vi "CM_FGV.vi"(7 "FGV_mods":T1=enum."Pulse", 8 "Error In":errorcluster, 11 "DataIn":variant) -> (0 "Error Out":errorcluster, 3 "Rotações":dbl[](array[numeric]))   [LabVIEW 2016]
uses:
  CM_mods.ctl
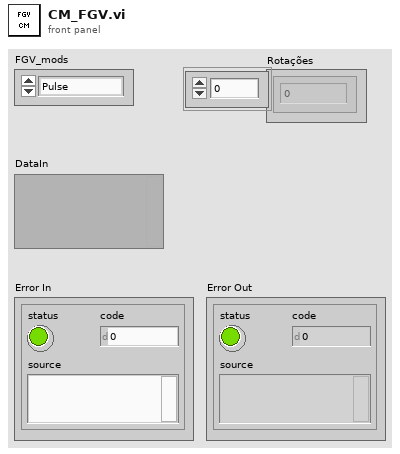
[diagram p1: front panel]
types:
  T1 = typedef "CM_mods.ctl" = enum16{"Init", "Pulse", "Retrieve", "End"}
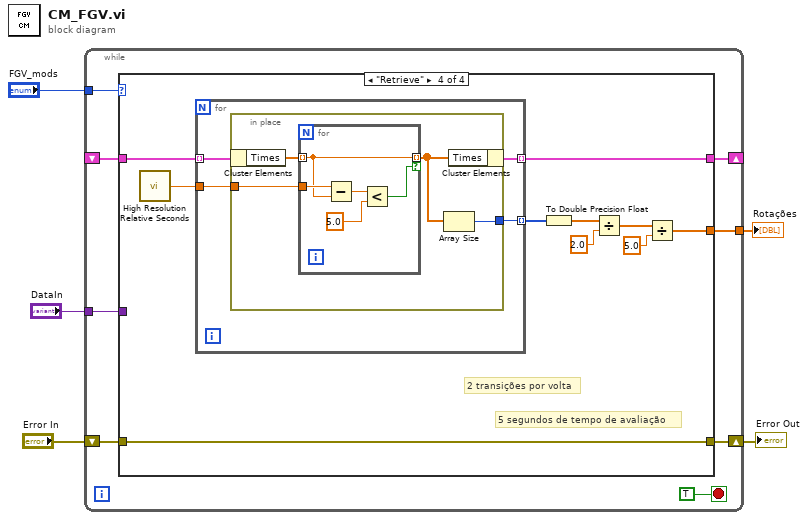
[diagram p0: block diagram]
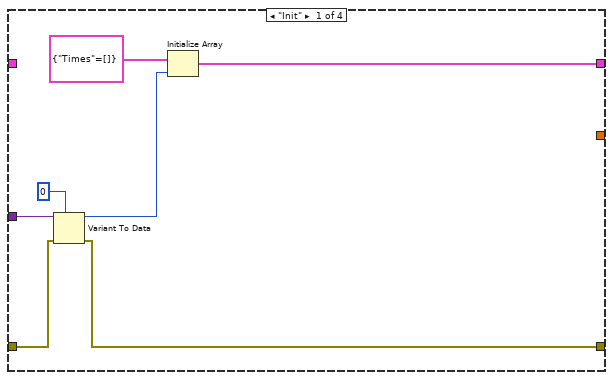
[diagram p2: hidden frame]
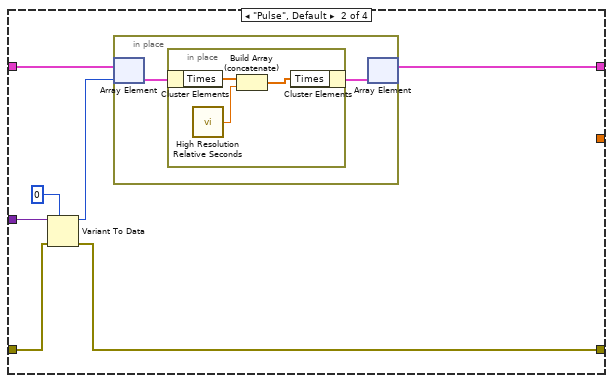
[diagram p3: hidden frame]
diagram:
  n1 = while {
    tunnel: "DataIn" -> [w12]
    tunnel: "FGV_mods" -> [w11]
    shift-right: [w10] -> _
    shift-left: _ -> [w9]
    shift-right: [w7] -> w2
    shift-left: "Error In" -> [w8]
    tunnel: [w6] -> w1
    stop <- TRUE stop-if-true
    n2 = case shown="\"Retrieve\"" w11 {
      tunnel: w12 -> [w20 w26 _ _]
      tunnel: [w16 w21 w34 w42] -> w10
      tunnel: w9 -> [_ w23 w34 w44]
      tunnel: w8 -> [w19 w25 w33 w35]
      tunnel: [w15 w24 w33 w35] -> w7
      tunnel: [_ _ _ w36] -> w6
      frame "Init" {
        n3 = Variant To Data(error in=w19, type=0, Variant=w20) -> (data=w17:i32, error out=w15:errorcluster)
        n4 = Initialize Array(cluster{"Times":dbl[]} {"Times"=[]}, w17) -> (w16:cluster{"Times":dbl[]}[])
      }
      frame "Pulse", Default {
        n5 = Variant To Data(error in=w25, type=0, Variant=w26) -> (data=w22:i32, error out=w24:errorcluster)
        n6 = in-place {
          n7 = in-place-array #1(w23, w22) -> (w29:cluster{"Times":dbl[]})
          n8 = in-place {
            n9 = in-place-cluster #2(w29) -> ("Times"=w32:dbl[])
            n10 = call <vilib>:"High Resolution Relative Seconds.vi"() -> ("relative seconds"=w31:dbl)
            n11 = Build Array (concatenate)(w32, w31) -> (w30:dbl[])
            n12 = in-place-cluster #2("Times"=w30) -> (w28:cluster{"Times":dbl[]})
          }
          n13 = in-place-array #1(w28) -> (w21:cluster{"Times":dbl[]}[])  [unwired: 1 out]
        }
      }
      frame "End" {
      }
      frame "Retrieve" {
        # "5 segundos de tempo de avaliação"
        # "2 transições por volta"
        n14 = call <vilib>:"High Resolution Relative Seconds.vi"() -> ("relative seconds"=w43:dbl)
        n15 = for {
          tunnel: w44 -> [w48] mode=indexing
          tunnel: w43 -> [w47]
          tunnel: [w46] -> w42 mode=indexing
          tunnel: [w45] -> w41 mode=indexing
          n16 = in-place {
            in-place-border: w47 -> [w51]
            in-place-border: [w49] -> w45
            n17 = in-place-cluster #3(w48) -> ("Times"=w52:dbl[])
            n18 = for {
              tunnel: w52 -> [w54] mode=indexing
              tunnel: w51 -> [w57]
              tunnel: [w54] -> w50 mode=indexing if=w53
              n19 = Subtract(x=w57, y=w54) -> (x-y=w56:dbl)
              n20 = Less?(x=w56, y=5.0) -> (x < y?=w53:bool)
            }
            n21 = Array Size(array=w50) -> (size(s)=w49:i32)
            n22 = in-place-cluster #3("Times"=w50) -> (w46:cluster{"Times":dbl[]})
          }
        }
        n23 = To Double Precision Float(number=w41) -> (double precision float=w40:dbl[])
        n24 = Divide(x=w40, y=2.0) -> (x/y=w37:dbl[])
        n25 = Divide(x=w37, y=5.0) -> (x/y=w36:dbl[])
      }
    }
  }
  "Error Out" <- w2
  "Rotações" <- w1
